vi "LOGIN.vi"() -> ()   [LabVIEW 2020]
uses:
  <vilib>/Utility/file.llb/Read Delimited Spreadsheet (string).vi
  <vilib>/Utility/file.llb/Write Delimited Spreadsheet (string).vi
panel:
  in  "Tab control 2":T1(tab)
  in  "Avanzar 2":bool
  in  "LOGIN 2":bool
  in  "CONTRASEÑA 2":string
  in  "USUARIO  2":string
  in  "Usuario a eliminar 2":string
  in  "Usuario nuevo 2":string
  in  "Contraseña nueva 2":string
  in  "Agregar usuario 2":bool
  in  "Terminar sesión admin 2":bool
  in  "Eliminar usuario 2":bool
  out "Base de datos 2":string[][](array[string])=[["Sabastian", "1234"], ["Fabio", "4321"], ["Keimer", "qwer"], ["Jorge", "0987"]]
  in  "Menu2":enum32{"1", "2", "3", "4", "5", "6"}(tab)
  out "Led8 2":bool
  out "Led7 2":bool
  out "Led6 2":bool
  out "Led5 2":bool
  out "Led4 2":bool
  out "Led3 2":bool
  out "Led2 2":bool
  out "Led1 2":bool
  out "Gráfica del seno 2":cluster{dbl[], dbl[]}(graph)
  out "Circulo de muerte 2":cluster{dbl[], dbl[]}(graph)
  out "tanque de chamber":dbl(slide) scale=0.0..100.0
  out "Fecha 2":string
  out "Hora 2":string
  out "Mensaje de bienvenida 2":string
  in  "Hora y fecha actual 2":bool
  in  "Llenado de un tanque 2":bool
  in  "Circulo de la muerte 2":bool
  in  "Gráfica del seno 2":bool
  in  "Secuencia de leds 2":bool
  in  "Terminar sesión usuario 2":bool
  in  "Tab control 1":T1(tab)
  in  "Avanzar":bool
  in  "LOGIN":bool
  in  "CONTRASEÑA":string
  in  "USUARIO":string
  in  "Usuario a eliminar":string
  in  "Usuario nuevo":string
  in  "Contraseña nueva":string
  in  "Agregar usuario":bool
  in  "Terminar sesión admin":bool
  in  "Eliminar usuario":bool
  out "Base de datos":string[][](array[string])=[["Sabastian", "1234"], ["Fabio", "4321"], ["Keimer", "qwer"], ["Jorge", "0987"]]
  in  "MenuU":enum32{"1", "2", "3", "4", "5", "6"}(tab)
  out "Led8":bool
  out "Led7":bool
  out "Led6":bool
  out "Led5":bool
  out "Led4":bool
  out "Led3":bool
  out "Led2":bool
  out "Led1":bool
  out "Gráfica del seno":cluster{dbl[], dbl[]}(graph)
  out "Circulo de muerte":cluster{dbl[], dbl[]}(graph)
  out "tanque de chamber":dbl(slide) scale=0.0..100.0
  out "Fecha":string
  out "Hora":string
  out "Mensaje de bienvenida":string
  in  "Hora actual y la fehca":bool
  in  "Llenado de un tanque":bool
  in  "Circulo de la muete":bool
  in  "Gráfica del seno":bool
  in  "Secuencia de leds":bool
  in  "Terminar sesión usuario":bool
  # "Bienvenidos"
  # "Fabio Alberto Figueroa Benitez\n\nNatalia Arenas Londoño\n\nLOGIN"
  # "Página principal"
  # "FYN SERVICES"
  # "LOGIN"
  # "Menú del administrador"
  # "Usuarios"
  # "Contraseñas"
  # "Secuencia de un leds"
  # "Llenado de un tanque chamber"
  # "Hora y fecha actual"
  # "Fecha"
  # "Hora"
  # "Bienvenidos"
  # "Fabio Alberto Figueroa Benitez\n\nNatalia Arenas Londoño\n\nLOGIN"
  # "Página principal"
  # "FYN SERVICES"
  # "LOGIN"
  # "Menú del administrador"
  # "Usuarios"
  # "Contraseñas"
  # "Secuencia de un leds"
  # "Llenado de un tanque chamber"
  # "Hora y fecha actual"
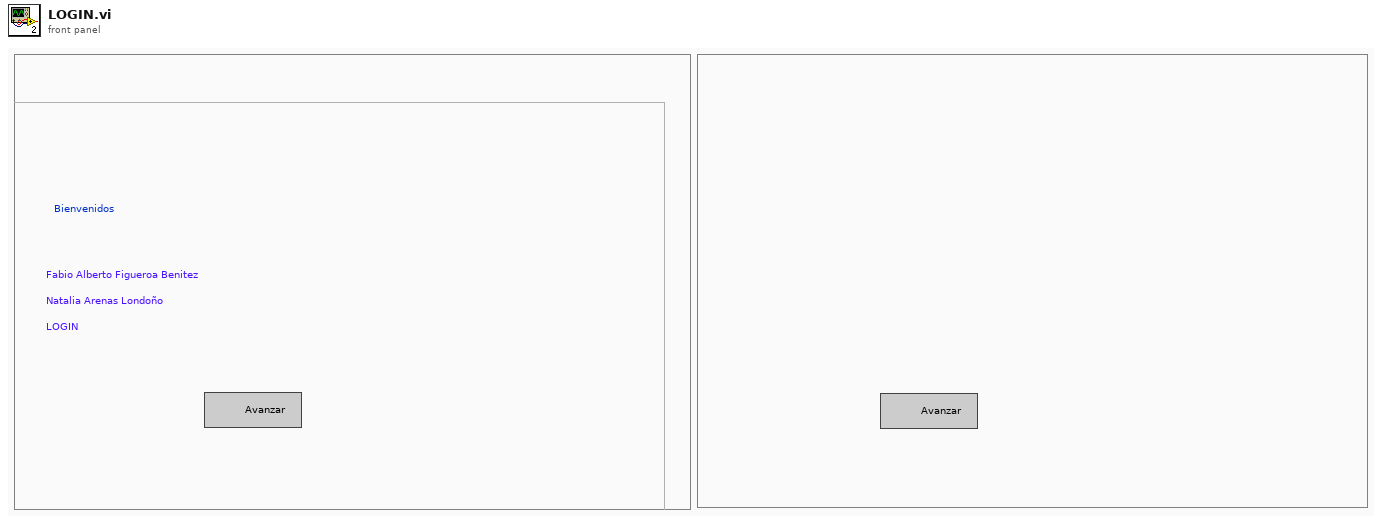
[diagram p1: front panel]
types:
  T1 = enum32{"Bienvenidos", "Principal", "Menú de administrador ", "Menú Usuario"}
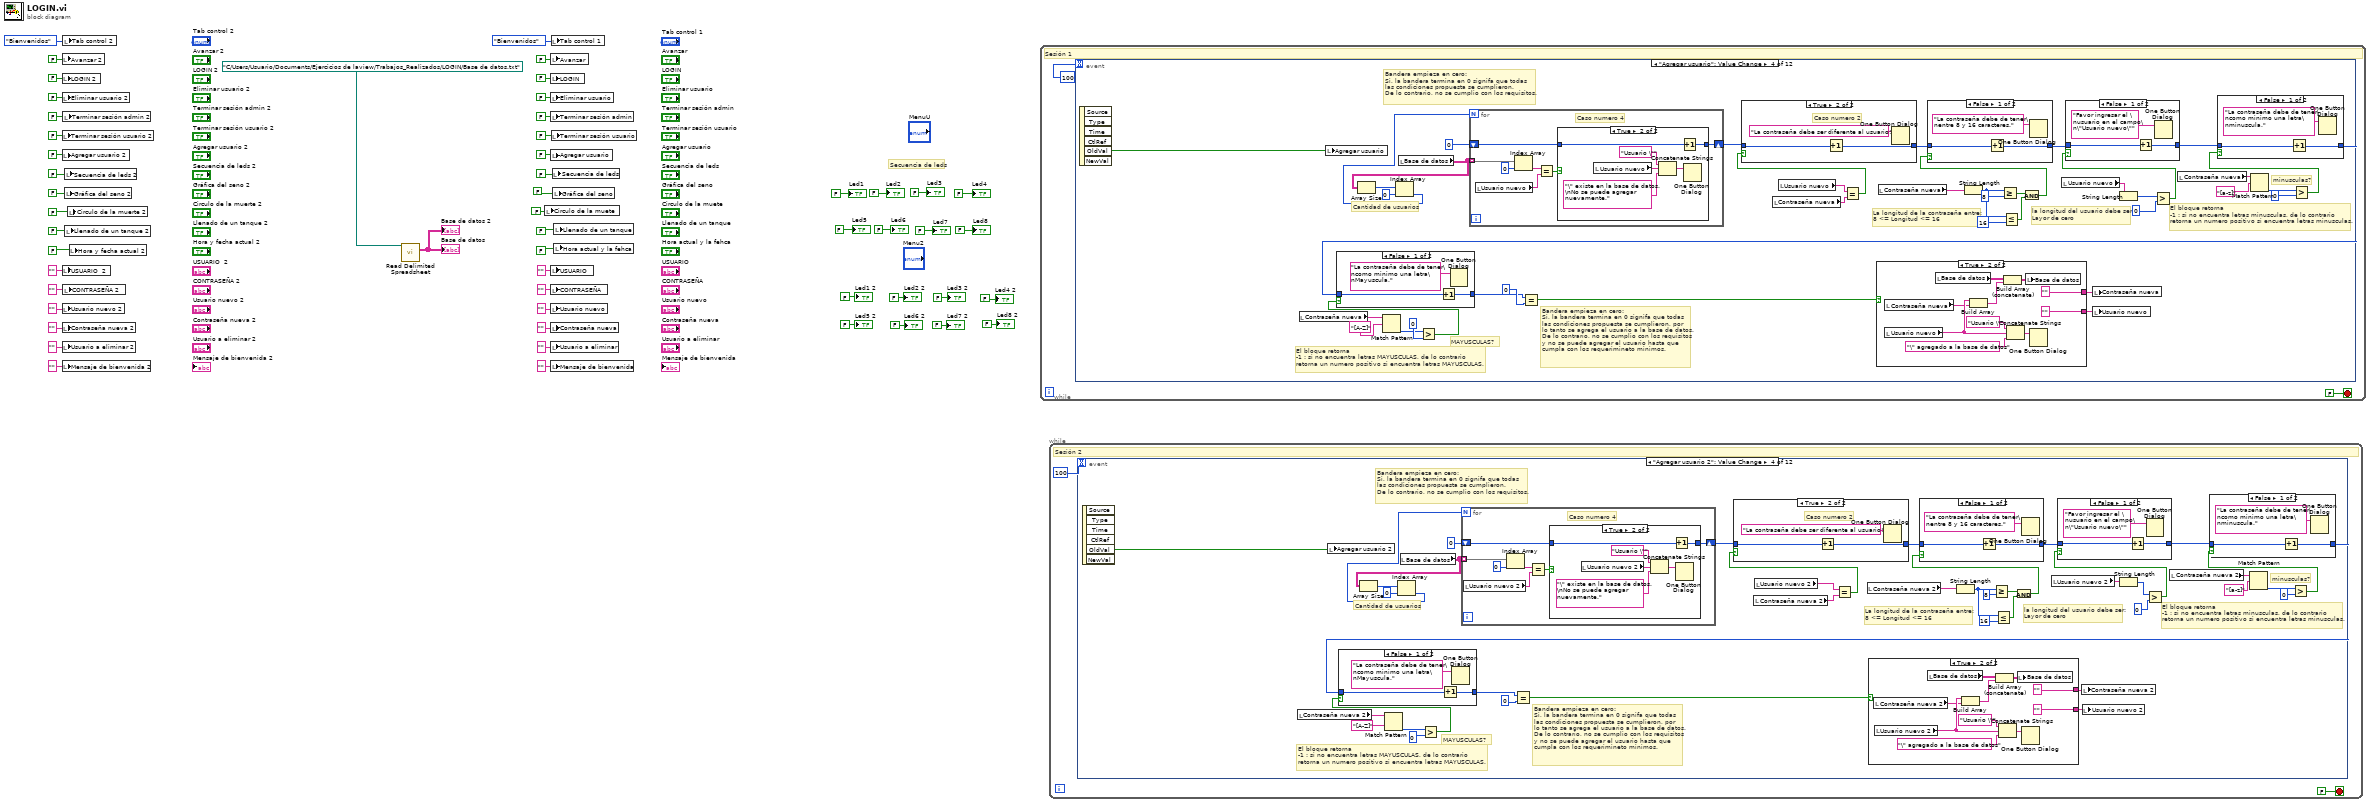
[diagram p0: block diagram]
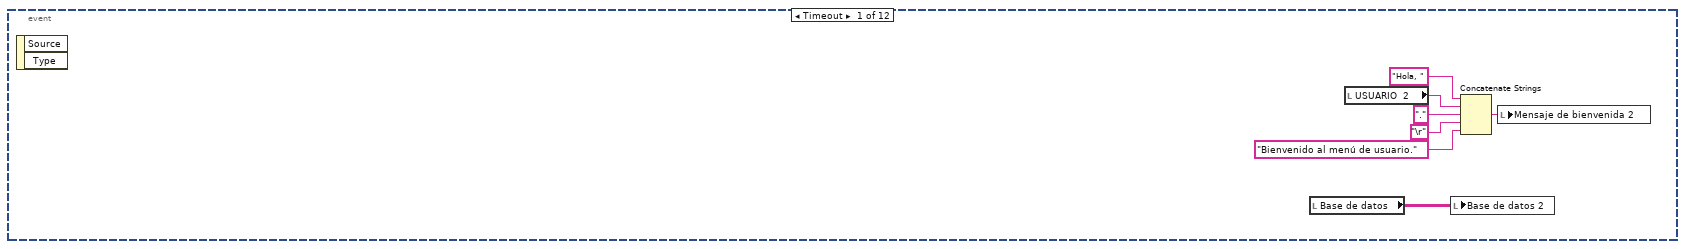
[diagram p2: hidden frame]
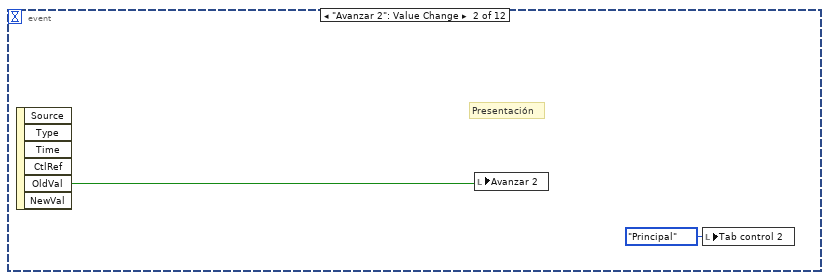
[diagram p3: hidden frame]
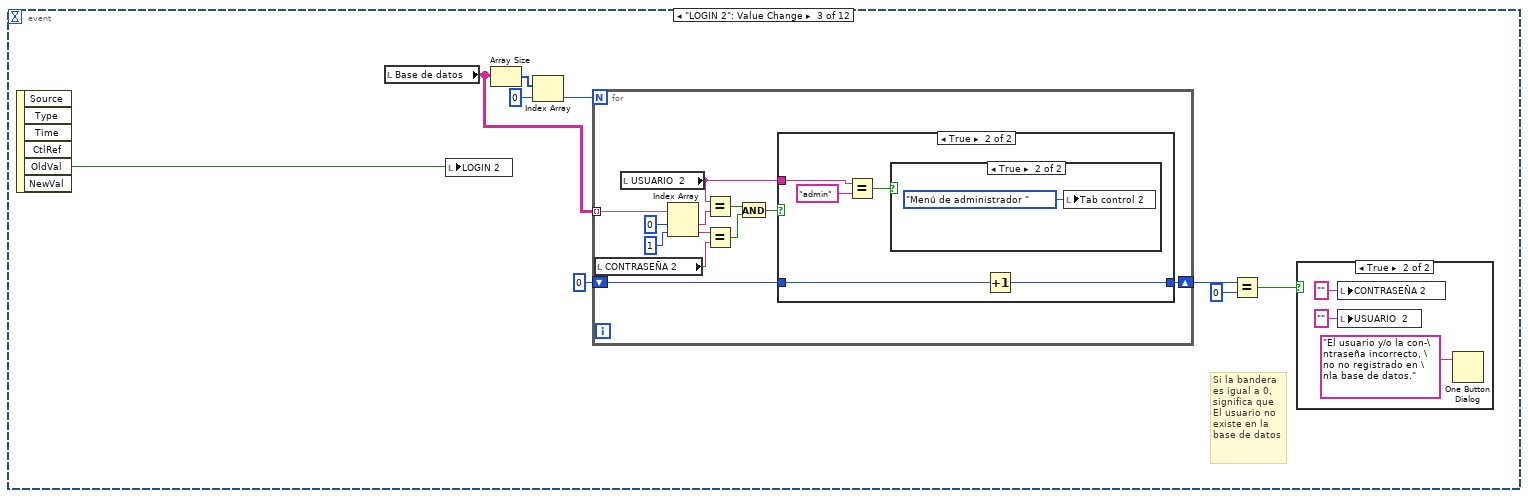
[diagram p4: hidden frame]
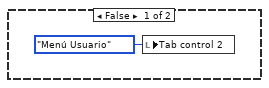
[diagram p7: hidden frame]
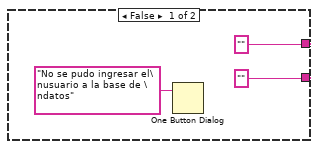
[diagram p8: hidden frame]
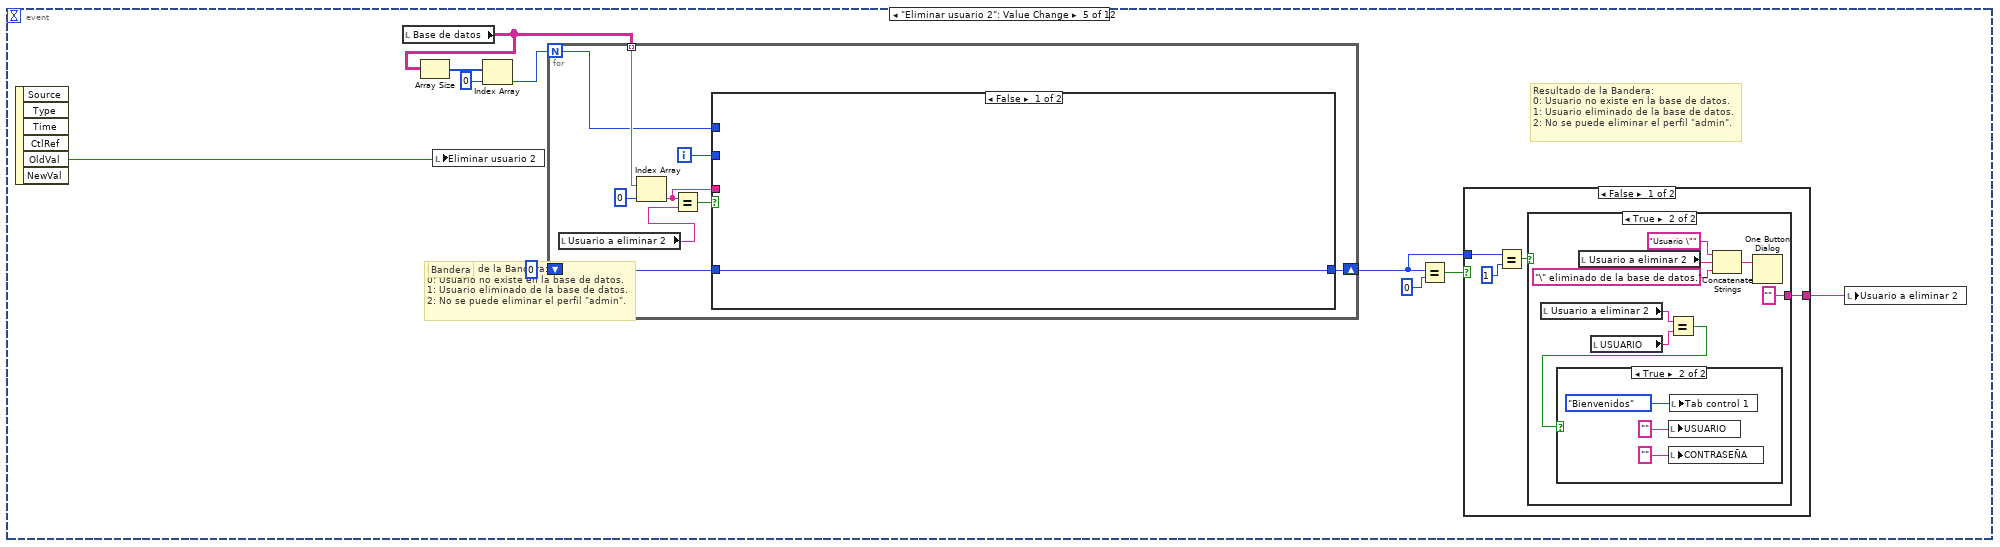
[diagram p15: hidden frame]
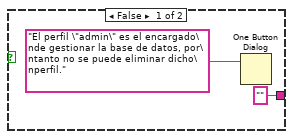
[diagram p16: hidden frame]
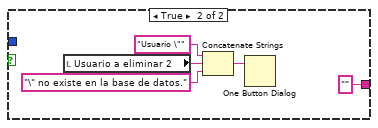
[diagram p18: hidden frame]
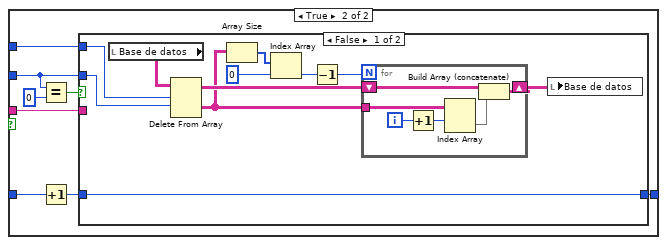
[diagram p19: hidden frame]
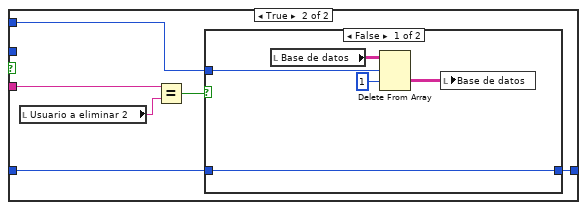
[diagram p20: hidden frame]
diagram:
  # "Secuencia de leds"
  n1 = local write "Avanzar 2"(FALSE ("Avanzar 2")) -> ()
  n2 = local write "LOGIN 2"(FALSE ("LOGIN 2")) -> ()
  n3 = local write "Eliminar usuario 2"(FALSE ("Eliminar usuario 2")) -> ()
  n4 = local write "Terminar sesión usuario 2"(FALSE ("Terminar sesión usuario 2")) -> ()
  n5 = local write "Agregar usuario 2"(FALSE ("Agregar usuario 2")) -> ()
  n6 = local write "USUARIO  2"("" ("USUARIO  2")) -> ()
  n7 = local write "Usuario nuevo 2"("" ("Usuario nuevo 2")) -> ()
  n8 = local write "Contraseña nueva 2"("" ("Contraseña nueva 2")) -> ()
  n9 = local write "Usuario a eliminar 2"("" ("Usuario a eliminar 2")) -> ()
  n10 = local write "Mensaje de bienvenida 2"("" ("Mensaje de bienvenida 2")) -> ()
  n11 = local write "Tab control 2"(T1."Bienvenidos" ("Tab control 2")) -> ()
  n12 = local write "Terminar sesión admin 2"(FALSE ("Terminar sesión admin 2")) -> ()
  n13 = local write "CONTRASEÑA 2"("" ("CONTRASEÑA 2")) -> ()
  n14 = local write "Secuencia de leds 2"(FALSE ("Luces de velocidad variable 2")) -> ()
  n15 = local write "Gráfica del seno 2"(FALSE ("Secuencia de LED 2")) -> ()
  n16 = local write "Llenado de un tanque 2"(FALSE ("Rutina 4 2")) -> ()
  n17 = local write "Circulo de la muerte 2"(FALSE ("Rutina 3 2")) -> ()
  n18 = local write "Hora y fecha actual 2"(FALSE ("Rutina 5 2")) -> ()
  n19 = call-poly <vilib>:"Read Delimited Spreadsheet.vi"("file path (dialog if empty)"=path "C:/Users/Usuario/Documents/Ejercicios de laview/Trabajos_Realizados/LOGIN/Base de datos.txt") -> ("all rows"=→"Base de datos" →"Base de datos 2":string[][])  [unwired: 9 in, 5 out]
  n20 = local write "Circulo de la muete"(FALSE ("Rutina 3")) -> ()
  n21 = local write "Avanzar"(FALSE ("Avanzar")) -> ()
  n22 = local write "LOGIN"(FALSE ("LOGIN")) -> ()
  n23 = local write "Eliminar usuario"(FALSE ("Eliminar usuario")) -> ()
  n24 = local write "Terminar sesión admin"(FALSE ("Terminar sesión admin")) -> ()
  n25 = local write "Agregar usuario"(FALSE ("Agregar usuario")) -> ()
  n26 = local write "USUARIO"("" ("USUARIO")) -> ()
  n27 = local write "CONTRASEÑA"("" ("CONTRASEÑA")) -> ()
  n28 = local write "Usuario nuevo"("" ("Usuario nuevo")) -> ()
  n29 = local write "Contraseña nueva"("" ("Contraseña nueva")) -> ()
  n30 = local write "Usuario a eliminar"("" ("Usuario a eliminar")) -> ()
  n31 = local write "Mensaje de bienvenida"("" ("Mensaje de bienvenida")) -> ()
  n32 = local write "Tab control 1"(T1."Bienvenidos" ("Tab control 1")) -> ()
  n33 = local write "Terminar sesión usuario"(FALSE ("Terminar sesión usuario")) -> ()
  n34 = local write "Secuencia de leds"(FALSE ("Luces de velocidad variable")) -> ()
  n35 = local write "Gráfica del seno"(FALSE ("Secuencia de LED")) -> ()
  n36 = local write "Llenado de un tanque"(FALSE ("Rutina 4")) -> ()
  n37 = local write "Hora actual y la fehca"(FALSE ("Rutina 5")) -> ()
  n38 = while {
    stop <- FALSE stop-if-true
    # "Sesión 1"
    n39 = event shown="[3] \"Agregar usuario\": Value Change" {
      selector: _ -> [_ _ _ _ _ _ _ _ _ _ _ _]
      dyn-events: _ -> [_ _ _ _ _ _ _ _ _ _ _ _]
      timeout: 100 -> [_ _ _ _ _ _ _ _ _ _ _ _]
      event Timeout {
        n40 = event-data() -> ()  [unwired: 1 in, 2 out]
        n41 = local read "Base de datos"() -> (w58:string[][])
        n42 = call-poly <vilib>:"Write Delimited Spreadsheet.vi"("file path (dialog if empty)"=path "C:/Users/Usuario/Documents/Ejercicios de laview/Trabajos_Realizados/LOGIN/Base de datos.txt", "2D data"=w58, "append to file? (new file:F)"=FALSE) -> ()  [unwired: 11 in, 2 out]
        n43 = local read "USUARIO"() -> (w64:string)
        n44 = Concatenate Strings("Hola, ", w64, ".", "\r", "Bienvenido al menú de usuario.") -> (w62:string)
        n45 = local write "Mensaje de bienvenida"(w62) -> ()
      }
      event "Avanzar": Value Change {
        # "Presentación"
        n46 = event-data() -> ("OldVal"=w66:bool)  [unwired: 1 in, 5 out]
        n47 = local write "Avanzar"(w66) -> ()
        n48 = local write "Tab control 1"(T1."Principal" ("Tab control")) -> ()
      }
      event "LOGIN": Value Change {
        # "Si la bandera \nes igual a 0,\nsignifica que\nEl usuario no \nexiste en la \nbase de datos"
        n49 = event-data() -> ("OldVal"=w76:bool)  [unwired: 1 in, 5 out]
        n50 = local write "LOGIN"(w76) -> ()
        n51 = local read "Base de datos"() -> (w72:string[][])
        n52 = Array Size(array=w72) -> (size(s)=w74:i32[])
        n53 = Index Array(array=w74, index=0) -> (element=w73:i32)
        n54 = for {
          N: w73 -> [_]
          tunnel: w72 -> [w91] mode=indexing
          shift-right: [w80] -> w70
          shift-left: 0 -> [w81]
          n55 = local read "CONTRASEÑA"() -> (w86:string)
          n56 = local read "USUARIO"() -> (w82:string)
          n57 = Index Array(array=w91, index #1=0 ("index"), index #2=1 ("index")) -> (element #1=w88:string, element #2=w87:string)
          n58 = Equal?(x=w82, y=w88) -> (x = y?=w85:bool)
          n59 = Equal?(x=w87, y=w86) -> (x = y?=w84:bool)
          n60 = And(x=w85, y=w84) -> (x .and. y?=w83:bool)
          n61 = case shown="True" w83 {
            tunnel: w82 -> [_ w97]
            tunnel: w81 -> [w92 w94]
            tunnel: [w92 w93] -> w80
            frame False {
            }
            frame True {
              n62 = Equal?(x=w97, y="admin") -> (x = y?=w95:bool)
              n63 = case shown="False" w95 {
                frame False {
                  n64 = local write "Tab control 1"(T1."Menú Usuario" ("Tab control")) -> ()
                }
                frame True {
                  n65 = local write "Tab control 1"(T1."Menú de administrador " ("Tab control")) -> ()
                }
              }
              n66 = Increment(x=w94) -> (x+1=w93:i32)
            }
          }
        }
        n67 = Equal?(x=w70, y=0) -> (x = y?=w68:bool)
        n68 = case shown="True" w68 {
          frame False {
          }
          frame True {
            n69 = local write "CONTRASEÑA"("") -> ()
            n70 = local write "USUARIO"("") -> ()
            n71 = One Button Dialog(message="El usuario y/o la con-\ntraseña incorrecto, \no no registrado en \nla base de datos.") -> ()  [unwired: 1 in, 1 out]
          }
        }
      }
      event "Agregar usuario": Value Change {
        # "Bandera empieza en cero:\nSi, la bandera termina en 0 signifa que todas \nlas condiciones propuesta se cumplieron, por \nlo tanto se agrega el usuario a la base de datos.\nDe lo contrario, no se cumplio con los requisitos\ny no se puede agregar el usuario hasta que \ncumpla con los requerimineto minimos."
        # "MAYUSCULAS?"
        # "El bloque retorna \n-1 : si no encuentra letras MAYUSCULAS, de lo contrario\nretorna un numero positivo si encuentra letras MAYUSCULAS."
        # "minusculas?"
        # "El bloque retorna \n-1 : si no encuentra letras minusculas, de lo contrario\nretorna un numero positivo si encuentra letras minusculas."
        # "la longitud del usuario debe ser:\nLayor de cero"
        # "La longitud de la contraseña entre:\n8 <= Longitud <= 16"
        # "Cantidad de usuarios"
        # "Bandera empieza en cero:\nSi, la bandera termina en 0 signifa que todas \nlas condiciones propuesta se cumplieron.\nDe lo contrario, no se cumplio con los requisitos."
        n72 = event-data() -> ("OldVal"=w139:bool)  [unwired: 1 in, 5 out]
        n73 = local read "Contraseña nueva"() -> (w107:string)
        n74 = local write "Agregar usuario"(w139) -> ()
        n75 = Match Pattern(string=w107, regular expression="[A-Z]") -> (offset past match=w110:i32)  [unwired: 1 in, 3 out]
        n76 = local read "Base de datos"() -> (w135:string[][])
        n77 = Array Size(array=w135) -> (size(s)=w137:i32[])
        n78 = Index Array(array=w137, index=0) -> (element=w134:i32)
        n79 = Greater?(x=w110, y=0) -> (0:w106:bool)
        n80 = for {
          N: w134 -> [_]
          tunnel: w135 -> [w178] mode=indexing
          shift-right: [w173] -> w131
          shift-left: 0 -> [w174]
          # "Caso numero 4"
          n81 = local read "Usuario nuevo"() -> (w176:string)
          n82 = Index Array(array=w178, index=0) -> (element=w177:string)
          n83 = Equal?(x=w177, y=w176) -> (x = y?=w175:bool)
          n84 = case shown="True" w175 {
            tunnel: w174 -> [w180 w182]
            tunnel: [w180 w181] -> w173
            frame False {
            }
            frame True {
              n85 = local read "Usuario nuevo"() -> (w183:string)
              n86 = Concatenate Strings("Usuario \"", w183, "\" existe en la base de datos.\nNo se puede agregar nuevamente." ("message")) -> (w185:string)
              n87 = Increment(x=w182) -> (x+1=w181:i32)
              n88 = One Button Dialog(message=w185) -> ()  [unwired: 1 in, 1 out]
            }
          }
        }
        n89 = local read "Contraseña nueva"() -> (w133:string)
        n90 = local read "Usuario nuevo"() -> (w132:string)
        n91 = Equal?(x=w132, y=w133) -> (x = y?=w100:bool)
        n92 = case shown="True" w100 {
          tunnel: w131 -> [w169 w170]
          tunnel: [w169 w171] -> w126
          frame False {
          }
          frame True {
            # "Caso numero 2"
            n93 = Increment(x=w170) -> (x+1=w171:i32)
            n94 = One Button Dialog(message="La contraseña debe ser diferente al usuario!") -> ()  [unwired: 1 in, 1 out]
          }
        }
        n95 = local read "Contraseña nueva"() -> (w124:string)
        n96 = String Length(string=w124) -> (length=w125:i32)
        n97 = Greater Or Equal?(x=w125, y=8) -> (x >= y?=w128:bool)
        n98 = Less Or Equal?(x=w125, y=16) -> (x <= y?=w127:bool)
        n99 = And(x=w128, y=w127) -> (x .and. y?=w123:bool)
        n100 = case shown="False" w123 {
          tunnel: w126 -> [w165 w168]
          tunnel: [w167 w168] -> w120
          frame False {
            n101 = Increment(x=w165) -> (x+1=w167:i32)
            n102 = One Button Dialog(message="La contraseña debe de tener\nentre 8 y 16 caracteres.") -> ()  [unwired: 1 in, 1 out]
          }
          frame True {
          }
        }
        n103 = local read "Usuario nuevo"() -> (w119:string)
        n104 = String Length(string=w119) -> (length=w122:i32)
        n105 = Greater?(x=w122, y=0) -> (0:w118:bool)
        n106 = case shown="False" w118 {
          tunnel: w120 -> [w163 w164]
          tunnel: [w162 w164] -> w114
          frame False {
            n107 = Increment(x=w163) -> (x+1=w162:i32)
            n108 = One Button Dialog(message="Favor ingresar el \nusuario en el campo\n\"Usuario nuevo\"") -> ()  [unwired: 1 in, 1 out]
          }
          frame True {
          }
        }
        n109 = local read "Contraseña nueva"() -> (w112:string)
        n110 = Match Pattern(string=w112, regular expression="[a-z]") -> (offset past match=w116:i32)  [unwired: 1 in, 3 out]
        n111 = Greater?(x=w116, y=0) -> (0:w113:bool)
        n112 = case shown="False" w113 {
          tunnel: w114 -> [w157 w160]
          tunnel: [w159 w160] -> w108
          frame False {
            n113 = Increment(x=w157) -> (x+1=w159:i32)
            n114 = One Button Dialog(message="La contraseña debe de tener\ncomo minimo una letra\nminuscula.") -> ()  [unwired: 1 in, 1 out]
          }
          frame True {
          }
        }
        n115 = case shown="False" w106 {
          tunnel: w108 -> [w153 w156]
          tunnel: [w155 w156] -> w104
          frame False {
            n116 = Increment(x=w153) -> (x+1=w155:i32)
            n117 = One Button Dialog(message="La contraseña debe de tener\ncomo minimo una letra\nMayuscula.") -> ()  [unwired: 1 in, 1 out]
          }
          frame True {
          }
        }
        n118 = Equal?(x=w104, y=0) -> (x = y?=w103:bool)
        n119 = case shown="True" w103 {
          tunnel: ["" ""] -> w102
          tunnel: ["" ""] -> w101
          frame False {
            n120 = One Button Dialog(message="No se pudo ingresar el\nusuario a la base de \ndatos") -> ()  [unwired: 1 in, 1 out]
          }
          frame True {
            n121 = local read "Contraseña nueva"() -> (w145:string)
            n122 = local read "Usuario nuevo"() -> (w146:string)
            n123 = local read "Base de datos"() -> (w147:string[][])
            n124 = Build Array(w146, w145) -> (w150:string[])
            n125 = Build Array (concatenate)(w147, w150) -> (w151:string[][])
            n126 = Concatenate Strings("Usuario \"", w146, "\" agregado a la base de datos" ("message")) -> (w152:string)
            n127 = local write "Base de datos"(w151) -> ()
            n128 = One Button Dialog(message=w152) -> ()  [unwired: 1 in, 1 out]
          }
        }
        n129 = local write "Contraseña nueva"(w102) -> ()
        n130 = local write "Usuario nuevo"(w101) -> ()
      }
      event "Eliminar usuario": Value Change {
        # "Resultado de la Bandera:\n0: Usuario no existe en la base de datos.\n1: Usuario eliminado de la base de datos.\n2: No se puede eliminar el perfil \"admin\"."
        # "Bandera"
        # "Resultado de la Bandera:\n0: Usuario no existe en la base de datos.\n1: Usuario eliminado de la base de datos.\n2: No se puede eliminar el perfil \"admin\"."
        n131 = event-data() -> ("OldVal"=w196:bool)  [unwired: 1 in, 5 out]
        n132 = local write "Eliminar usuario"(w196) -> ()
        n133 = local read "Base de datos"() -> (w192:string[][])
        n134 = Array Size(array=w192) -> (size(s)=w195:i32[])
        n135 = Index Array(array=w195, index=0) -> (element=w193:i32)
        n136 = for {
          N: w193 -> [w222]
          tunnel: w192 -> [w226] mode=indexing
          shift-right: [w220] -> w188
          shift-left: 0 -> [w221]
          i -> [w223]
          n137 = local read "Usuario a eliminar"() -> (w225:string)
          n138 = Index Array(array=w226, index=0) -> (element=w219:string)
          n139 = Equal?(x=w219, y=w225) -> (x = y?=w224:bool)
          n140 = case shown="True" w224 {
            tunnel: w223 -> [_ w233]
            tunnel: w222 -> [_ w234]
            tunnel: w221 -> [w228 w231]
            tunnel: [w228 w229] -> w220
            tunnel: w219 -> [_ w232]
            frame False {
            }
            frame True {
              n141 = Equal?(x=w233, y=0) -> (x = y?=w235:bool)
              n142 = Increment(x=w231) -> (x+1=w230:i32)
              n143 = case shown="False" w235 {
                tunnel: w234 -> [w243 w256]
                tunnel: w233 -> [w242 _]
                tunnel: w232 -> [_ w258]
                tunnel: w230 -> [w237 w255]
                tunnel: [w237 w254] -> w229
                frame False {
                  n144 = local read "Base de datos"() -> (w244:string[][])
                  n145 = Delete From Array(array=w244, length=w243, index (row)=w242) -> (deleted portion=w239:string[][], array with subset deleted=w240:string[][])  [unwired: 1 in]
                  n146 = Array Size(array=w239) -> (size(s)=w246:i32[])
                  n147 = Index Array(array=w246, index=0) -> (element=w245:i32)
                  n148 = Decrement(x=w245) -> (x-1=w241:i32)
                  n149 = for {
                    N: w241 -> [_]
                    shift-right: [w248] -> w238
                    shift-left: w240 -> [w252]
                    tunnel: w239 -> [w251]
                    i -> [w253]
                    n150 = Increment(x=w253) -> (x+1=w250:i32)
                    n151 = Index Array(array=w251, index (row)=w250) -> (element=w249:string[])  [unwired: 1 in]
                    n152 = Build Array (concatenate)(w252, w249) -> (w248:string[][])
                  }
                  n153 = local write "Base de datos"(w238) -> ()
                }
                frame True {
                  n154 = local read "Usuario a eliminar"() -> (w259:string)
                  n155 = Equal?(x=w258, y=w259) -> (x = y?=w257:bool)
                  n156 = case shown="True" w257 {
                    tunnel: w256 -> [w261 _]
                    tunnel: w255 -> [w260 w266]
                    tunnel: [w260 w265] -> w254
                    frame False {
                      n157 = local read "Base de datos"() -> (w264:string[][])
                      n158 = Delete From Array(array=w264, length=w261, index (row)=1) -> (deleted portion=w263:string[][])  [unwired: 1 in, 1 out]
                      n159 = local write "Base de datos"(w263) -> ()
                    }
                    frame True {
                      n160 = Increment(x=w266) -> (x+1=w265:i32)
                      n161 = One Button Dialog(message="No se puede eliminar el perfir de \"admin\".") -> ()  [unwired: 1 in, 1 out]
                    }
                  }
                }
              }
            }
          }
        }
        n162 = Equal?(x=w188, y=0) -> (x = y?=w189:bool)
        n163 = case shown="False" w189 {
          tunnel: w188 -> [w199 _]
          tunnel: [w197 ""] -> w187
          frame False {
            n164 = Equal?(x=w199, y=1) -> (x = y?=w200:bool)
            n165 = case shown="True" w200 {
              tunnel: ["" ""] -> w197
              frame False {
                n166 = One Button Dialog(message="El perfil \"admin\" es el encargado\nde gestionar la base de datos, por\ntanto no se puede eliminar dicho\nperfil.") -> ()  [unwired: 1 in, 1 out]
              }
              frame True {
                n167 = local read "Usuario a eliminar"() -> (w204:string)
                n168 = local read "USUARIO  2"() -> (w205:string)
                n169 = local read "Usuario a eliminar"() -> (w209:string)
                n170 = Equal?(x=w204, y=w205) -> (x = y?=w203:bool)
                n171 = case shown="True" w203 {
                  frame False {
                  }
                  frame True {
                    n172 = local write "USUARIO  2"("") -> ()
                    n173 = local write "Tab control 2"(T1."Bienvenidos" ("Tab control")) -> ()
                    n174 = local write "CONTRASEÑA 2"("") -> ()
                  }
                }
                n175 = Concatenate Strings("Usuario \"", w209, "\" eliminado de la base de datos." ("message")) -> (w210:string)
                n176 = One Button Dialog(message=w210) -> ()  [unwired: 1 in, 1 out]
              }
            }
          }
          frame True {
            n177 = local read "Usuario a eliminar"() -> (w215:string)
            n178 = Concatenate Strings("Usuario \"", w215, "\" no existe en la base de datos." ("message")) -> (w218:string)
            n179 = One Button Dialog(message=w218) -> ()  [unwired: 1 in, 1 out]
          }
        }
        n180 = local write "Usuario a eliminar"(w187) -> ()
      }
      event "Terminar sesión admin": Value Change {
        n181 = event-data() -> ("OldVal"=w271:bool)  [unwired: 1 in, 5 out]
        n182 = local write "Terminar sesión admin"(w271) -> ()
        n183 = local write "Tab control 1"(T1."Bienvenidos" ("Tab control")) -> ()
        n184 = local write "USUARIO"("") -> ()
        n185 = local write "CONTRASEÑA"("") -> ()
      }
      event "Terminar sesión usuario": Value Change {
        n186 = event-data() -> ("OldVal"=w272:bool)  [unwired: 1 in, 5 out]
        n187 = local write "Terminar sesión usuario"(w272) -> ()
        n188 = local write "Tab control 1"(T1."Bienvenidos" ("Tab control")) -> ()
        n189 = local write "USUARIO"("") -> ()
        n190 = local write "CONTRASEÑA"("") -> ()
      }
      event "Secuencia de leds": Value Change {
        # "Secuencia de leds"
        n191 = event-data() -> ("OldVal"=w277:bool)  [unwired: 1 in, 5 out]
        n192 = local write "Secuencia de leds"(w277) -> ()
        n193 = flat-sequence {
          frame #0 {
            n194 = local read "Led1"() -> (w280:bool)
            n195 = Not(x=w280) -> (.not. x?=w279:bool)
            n196 = Wait (ms)(milliseconds to wait=u32 1000) -> ()  [unwired: 1 out]
            n197 = local write "Led1"(w279) -> ()
          }
          frame #1 {
            n198 = local read "Led2"() -> (w282:bool)
            n199 = Wait (ms)(milliseconds to wait=u32 1000) -> ()  [unwired: 1 out]
            n200 = Not(x=w282) -> (.not. x?=w283:bool)
            n201 = local write "Led2"(w283) -> ()
            n202 = local write "Led1"(FALSE ("Led1")) -> ()
          }
          frame #2 {
            n203 = local read "Led3"() -> (w287:bool)
            n204 = Wait (ms)(milliseconds to wait=u32 1000) -> ()  [unwired: 1 out]
            n205 = Not(x=w287) -> (.not. x?=w286:bool)
            n206 = local write "Led3"(w286) -> ()
            n207 = local write "Led2"(FALSE ("Led1")) -> ()
          }
          frame #3 {
            n208 = local read "Led4"() -> (w291:bool)
            n209 = Wait (ms)(milliseconds to wait=u32 1000) -> ()  [unwired: 1 out]
            n210 = Not(x=w291) -> (.not. x?=w292:bool)
            n211 = local write "Led4"(w292) -> ()
            n212 = local write "Led3"(FALSE ("Led1")) -> ()
          }
          frame #4 {
            n213 = local read "Led5"() -> (w294:bool)
            n214 = Wait (ms)(milliseconds to wait=u32 1000) -> ()  [unwired: 1 out]
            n215 = Not(x=w294) -> (.not. x?=w293:bool)
            n216 = local write "Led5"(w293) -> ()
            n217 = local write "Led4"(FALSE ("Led1")) -> ()
          }
          frame #5 {
            n218 = local read "Led6"() -> (w299:bool)
            n219 = Wait (ms)(milliseconds to wait=u32 1000) -> ()  [unwired: 1 out]
            n220 = Not(x=w299) -> (.not. x?=w300:bool)
            n221 = local write "Led6"(w300) -> ()
            n222 = local write "Led5"(FALSE ("Led1")) -> ()
          }
          frame #6 {
            n223 = local read "Led7"() -> (w303:bool)
            n224 = Wait (ms)(milliseconds to wait=u32 1000) -> ()  [unwired: 1 out]
            n225 = Not(x=w303) -> (.not. x?=w302:bool)
            n226 = local write "Led7"(w302) -> ()
            n227 = local write "Led6"(FALSE ("Led1")) -> ()
          }
          frame #7 {
            n228 = local read "Led8"() -> (w306:bool)
            n229 = Wait (ms)(milliseconds to wait=u32 1000) -> ()  [unwired: 1 out]
            n230 = Not(x=w306) -> (.not. x?=w307:bool)
            n231 = local write "Led8"(w307) -> ()
            n232 = local write "Led7"(FALSE ("Led1")) -> ()
          }
          frame #8 {
            n233 = Wait (ms)(milliseconds to wait=u32 1000) -> ()  [unwired: 1 out]
            n234 = local write "Led8"(FALSE ("Led1")) -> ()
          }
        }
        n235 = local write "MenuU"(enum32{"1", "2", "3", "4", "5", "6"}."2" ("MenuU")) -> ()
      }
      event "Gráfica del seno": Value Change {
        # "Gráfica del seno"
        # "Este bloque\nrecibe un cluster"
        # "Para mostrar la gráfoca en x,  y"
        n236 = event-data() -> ("OldVal"=w311:bool)  [unwired: 1 in, 5 out]
        n237 = local write "MenuU"(enum32{"1", "2", "3", "4", "5", "6"}."3" ("MenuU")) -> ()
        n238 = local write "Gráfica del seno"(w311) -> ()
        n239 = Multiply(x=200.0, y=3.141592653589793) -> (x*y=w317:dbl)
        n240 = for {
          N: w317 -> [_]
          tunnel: [w320] -> w312 mode=indexing
          tunnel: [w319] -> w313 mode=indexing
          i -> [w323]
          # "x"
          # "y"
          n241 = Wait (ms)(milliseconds to wait=u32 1) -> ()  [unwired: 1 out]
          n242 = Divide(x=w323, y=100) -> (x/y=w319:dbl)
          n243 = Sine(x=w319) -> (sin(x)=w320:dbl)
        }
        n244 = Bundle(w313, w312) -> (→"Gráfica del seno":cluster{dbl[], dbl[]})  [unwired: 1 in]
      }
      event "Circulo de la muete": Value Change {
        n245 = event-data() -> ("OldVal"=w329:bool)  [unwired: 1 in, 5 out]
        n246 = local write "Circulo de la muete"(w329) -> ()
        n247 = for {
          N: 100 -> [_]
          tunnel: [w332] -> w327 mode=indexing
          tunnel: [w330] -> w326 mode=indexing
          i -> [w331]
          n248 = Multiply(x=0.3183098861837907, y=w331) -> (x*y=w334:dbl)
          n249 = Sine & Cosine(0:w334) -> (1:w333:dbl, 2:w330:dbl)
          n250 = Multiply(x=w333, y=w331) -> (x*y=w332:dbl)
        }
        n251 = local write "MenuU"(enum32{"1", "2", "3", "4", "5", "6"}."4" ("MenuU")) -> ()
        n252 = Bundle(w327, w326) -> (→"Circulo de muerte":cluster{dbl[], dbl[]})  [unwired: 1 in]
      }
      event "Llenado de un tanque": Value Change {
        n253 = event-data() -> ("OldVal"=w338:bool)  [unwired: 1 in, 5 out]
        n254 = local write "Llenado de un tanque"(w338) -> ()
        n255 = for {
          N: 100 -> [_]
          i -> [w340]
          n256 = Wait (ms)(milliseconds to wait=u32 100) -> ()  [unwired: 1 out]
          "tanque de chamber" <- w340
        }
        n257 = local write "MenuU"(enum32{"1", "2", "3", "4", "5", "6"}."5" ("MenuU")) -> ()
      }
      event "Hora actual y la fehca": Value Change {
        # "Hora"
        # "Fecha"
        n258 = event-data() -> ("OldVal"=w353:bool)  [unwired: 1 in, 5 out]
        n259 = local write "Hora actual y la fehca"(w353) -> ()
        n260 = Get Date/Time In Seconds() -> (seconds since 1Jan1904=w352:timestamp)
        n261 = Get Date/Time In Seconds() -> (seconds since 1Jan1904=w342:timestamp)
        n262 = local write "MenuU"(enum32{"1", "2", "3", "4", "5", "6"}."6" ("MenuU")) -> ()
        n263 = Get Date/Time String(seconds (now)=w352) -> (date string=w351:string)  [unwired: 2 in, 1 out]
        n264 = Get Date/Time String(seconds (now)=w342) -> (time string=w341:string)  [unwired: 2 in, 1 out]
        n265 = Concatenate Strings("Fecha:" ("date string"), "\n", "\n", w351) -> (→"Fecha":string)
        n266 = Concatenate Strings("Hora:" ("date string"), "\n", "\n", w341) -> (→"Hora":string)
      }
    }
  }
  n267 = while {
    stop <- FALSE stop-if-true
    # "Sesión 2"
    n268 = event shown="[3] \"Agregar usuario 2\": Value Change" {
      selector: _ -> [_ _ _ _ _ _ _ _ _ _ _ _]
      dyn-events: _ -> [_ _ _ _ _ _ _ _ _ _ _ _]
      timeout: 100 -> [_ _ _ _ _ _ _ _ _ _ _ _]
      event Timeout {
        n269 = event-data() -> ()  [unwired: 1 in, 2 out]
        n270 = local read "Base de datos"() -> (w357:string[][])
        n271 = local read "USUARIO  2"() -> (w362:string)
        n272 = local write "Base de datos 2"(w357) -> ()
        n273 = Concatenate Strings("Hola, ", w362, ".", "\r", "Bienvenido al menú de usuario.") -> (w360:string)
        n274 = local write "Mensaje de bienvenida 2"(w360) -> ()
      }
      event "Avanzar 2": Value Change {
        # "Presentación"
        n275 = event-data() -> ("OldVal"=w364:bool)  [unwired: 1 in, 5 out]
        n276 = local write "Avanzar 2"(w364) -> ()
        n277 = local write "Tab control 2"(T1."Principal" ("Tab control")) -> ()
      }
      event "LOGIN 2": Value Change {
        # "Si la bandera \nes igual a 0,\nsignifica que\nEl usuario no \nexiste en la \nbase de datos"
        n278 = event-data() -> ("OldVal"=w374:bool)  [unwired: 1 in, 5 out]
        n279 = local read "Base de datos"() -> (w370:string[][])
        n280 = local write "LOGIN 2"(w374) -> ()
        n281 = Array Size(array=w370) -> (size(s)=w372:i32[])
        n282 = Index Array(array=w372, index=0) -> (element=w371:i32)
        n283 = for {
          N: w371 -> [_]
          tunnel: w370 -> [w389] mode=indexing
          shift-right: [w378] -> w368
          shift-left: 0 -> [w379]
          n284 = local read "CONTRASEÑA 2"() -> (w384:string)
          n285 = local read "USUARIO  2"() -> (w380:string)
          n286 = Index Array(array=w389, index #1=0 ("index"), index #2=1 ("index")) -> (element #1=w386:string, element #2=w385:string)
          n287 = Equal?(x=w380, y=w386) -> (x = y?=w383:bool)
          n288 = Equal?(x=w385, y=w384) -> (x = y?=w382:bool)
          n289 = And(x=w383, y=w382) -> (x .and. y?=w381:bool)
          n290 = case shown="True" w381 {
            tunnel: w380 -> [_ w395]
            tunnel: w379 -> [w390 w392]
            tunnel: [w390 w391] -> w378
            frame False {
            }
            frame True {
              n291 = Equal?(x=w395, y="admin") -> (x = y?=w393:bool)
              n292 = case shown="True" w393 {
                frame False {
                  n293 = local write "Tab control 2"(T1."Menú Usuario" ("Tab control")) -> ()
                }
                frame True {
                  n294 = local write "Tab control 2"(T1."Menú de administrador " ("Tab control")) -> ()
                }
              }
              n295 = Increment(x=w392) -> (x+1=w391:i32)
            }
          }
        }
        n296 = Equal?(x=w368, y=0) -> (x = y?=w366:bool)
        n297 = case shown="True" w366 {
          frame False {
          }
          frame True {
            n298 = local write "CONTRASEÑA 2"("") -> ()
            n299 = local write "USUARIO  2"("") -> ()
            n300 = One Button Dialog(message="El usuario y/o la con-\ntraseña incorrecto, \no no registrado en \nla base de datos.") -> ()  [unwired: 1 in, 1 out]
          }
        }
      }
      event "Agregar usuario 2": Value Change {
        # "Bandera empieza en cero:\nSi, la bandera termina en 0 signifa que todas \nlas condiciones propuesta se cumplieron, por \nlo tanto se agrega el usuario a la base de datos.\nDe lo contrario, no se cumplio con los requisitos\ny no se puede agregar el usuario hasta que \ncumpla con los requerimineto minimos."
        # "MAYUSCULAS?"
        # "El bloque retorna \n-1 : si no encuentra letras MAYUSCULAS, de lo contrario\nretorna un numero positivo si encuentra letras MAYUSCULAS."
        # "minusculas?"
        # "El bloque retorna \n-1 : si no encuentra letras minusculas, de lo contrario\nretorna un numero positivo si encuentra letras minusculas."
        # "la longitud del usuario debe ser:\nLayor de cero"
        # "La longitud de la contraseña entre:\n8 <= Longitud <= 16"
        # "Cantidad de usuarios"
        # "Bandera empieza en cero:\nSi, la bandera termina en 0 signifa que todas \nlas condiciones propuesta se cumplieron.\nDe lo contrario, no se cumplio con los requisitos."
        n301 = event-data() -> ("OldVal"=w437:bool)  [unwired: 1 in, 5 out]
        n302 = local read "Contraseña nueva 2"() -> (w405:string)
        n303 = local write "Agregar usuario 2"(w437) -> ()
        n304 = Match Pattern(string=w405, regular expression="[A-Z]") -> (offset past match=w408:i32)  [unwired: 1 in, 3 out]
        n305 = local read "Base de datos"() -> (w433:string[][])
        n306 = Array Size(array=w433) -> (size(s)=w435:i32[])
        n307 = Index Array(array=w435, index=0) -> (element=w432:i32)
        n308 = Greater?(x=w408, y=0) -> (0:w404:bool)
        n309 = for {
          N: w432 -> [_]
          tunnel: w433 -> [w476] mode=indexing
          shift-right: [w471] -> w429
          shift-left: 0 -> [w472]
          # "Caso numero 4"
          n310 = local read "Usuario nuevo 2"() -> (w474:string)
          n311 = Index Array(array=w476, index=0) -> (element=w475:string)
          n312 = Equal?(x=w475, y=w474) -> (x = y?=w473:bool)
          n313 = case shown="True" w473 {
            tunnel: w472 -> [w478 w480]
            tunnel: [w478 w479] -> w471
            frame False {
            }
            frame True {
              n314 = local read "Usuario nuevo 2"() -> (w481:string)
              n315 = Concatenate Strings("Usuario \"", w481, "\" existe en la base de datos.\nNo se puede agregar nuevamente." ("message")) -> (w483:string)
              n316 = Increment(x=w480) -> (x+1=w479:i32)
              n317 = One Button Dialog(message=w483) -> ()  [unwired: 1 in, 1 out]
            }
          }
        }
        n318 = local read "Contraseña nueva 2"() -> (w431:string)
        n319 = local read "Usuario nuevo 2"() -> (w430:string)
        n320 = Equal?(x=w430, y=w431) -> (x = y?=w398:bool)
        n321 = case shown="True" w398 {
          tunnel: w429 -> [w467 w468]
          tunnel: [w467 w469] -> w424
          frame False {
          }
          frame True {
            # "Caso numero 2"
            n322 = Increment(x=w468) -> (x+1=w469:i32)
            n323 = One Button Dialog(message="La contraseña debe ser diferente al usuario!") -> ()  [unwired: 1 in, 1 out]
          }
        }
        n324 = local read "Contraseña nueva 2"() -> (w422:string)
        n325 = String Length(string=w422) -> (length=w423:i32)
        n326 = Greater Or Equal?(x=w423, y=8) -> (x >= y?=w426:bool)
        n327 = Less Or Equal?(x=w423, y=16) -> (x <= y?=w425:bool)
        n328 = And(x=w426, y=w425) -> (x .and. y?=w421:bool)
        n329 = case shown="False" w421 {
          tunnel: w424 -> [w463 w466]
          tunnel: [w465 w466] -> w418
          frame False {
            n330 = Increment(x=w463) -> (x+1=w465:i32)
            n331 = One Button Dialog(message="La contraseña debe de tener\nentre 8 y 16 caracteres.") -> ()  [unwired: 1 in, 1 out]
          }
          frame True {
          }
        }
        n332 = local read "Usuario nuevo 2"() -> (w417:string)
        n333 = String Length(string=w417) -> (length=w420:i32)
        n334 = Greater?(x=w420, y=0) -> (0:w416:bool)
        n335 = case shown="False" w416 {
          tunnel: w418 -> [w461 w462]
          tunnel: [w460 w462] -> w412
          frame False {
            n336 = Increment(x=w461) -> (x+1=w460:i32)
            n337 = One Button Dialog(message="Favor ingresar el \nusuario en el campo\n\"Usuario nuevo\"") -> ()  [unwired: 1 in, 1 out]
          }
          frame True {
          }
        }
        n338 = local read "Contraseña nueva 2"() -> (w410:string)
        n339 = Match Pattern(string=w410, regular expression="[a-z]") -> (offset past match=w414:i32)  [unwired: 1 in, 3 out]
        n340 = Greater?(x=w414, y=0) -> (0:w411:bool)
        n341 = case shown="False" w411 {
          tunnel: w412 -> [w455 w458]
          tunnel: [w457 w458] -> w406
          frame False {
            n342 = Increment(x=w455) -> (x+1=w457:i32)
            n343 = One Button Dialog(message="La contraseña debe de tener\ncomo minimo una letra\nminuscula.") -> ()  [unwired: 1 in, 1 out]
          }
          frame True {
          }
        }
        n344 = case shown="False" w404 {
          tunnel: w406 -> [w451 w454]
          tunnel: [w453 w454] -> w402
          frame False {
            n345 = Increment(x=w451) -> (x+1=w453:i32)
            n346 = One Button Dialog(message="La contraseña debe de tener\ncomo minimo una letra\nMayuscula.") -> ()  [unwired: 1 in, 1 out]
          }
          frame True {
          }
        }
        n347 = Equal?(x=w402, y=0) -> (x = y?=w401:bool)
        n348 = case shown="True" w401 {
          tunnel: ["" ""] -> w400
          tunnel: ["" ""] -> w399
          frame False {
            n349 = One Button Dialog(message="No se pudo ingresar el\nusuario a la base de \ndatos") -> ()  [unwired: 1 in, 1 out]
          }
          frame True {
            n350 = local read "Contraseña nueva 2"() -> (w443:string)
            n351 = local read "Usuario nuevo 2"() -> (w444:string)
            n352 = local read "Base de datos"() -> (w445:string[][])
            n353 = Build Array(w444, w443) -> (w448:string[])
            n354 = Build Array (concatenate)(w445, w448) -> (w449:string[][])
            n355 = Concatenate Strings("Usuario \"", w444, "\" agregado a la base de datos" ("message")) -> (w450:string)
            n356 = local write "Base de datos"(w449) -> ()
            n357 = One Button Dialog(message=w450) -> ()  [unwired: 1 in, 1 out]
          }
        }
        n358 = local write "Contraseña nueva 2"(w400) -> ()
        n359 = local write "Usuario nuevo 2"(w399) -> ()
      }
      event "Eliminar usuario 2": Value Change {
        # "Resultado de la Bandera:\n0: Usuario no existe en la base de datos.\n1: Usuario eliminado de la base de datos.\n2: No se puede eliminar el perfil \"admin\"."
        # "Bandera"
        # "Resultado de la Bandera:\n0: Usuario no existe en la base de datos.\n1: Usuario eliminado de la base de datos.\n2: No se puede eliminar el perfil \"admin\"."
        n360 = event-data() -> ("OldVal"=w494:bool)  [unwired: 1 in, 5 out]
        n361 = local read "Base de datos"() -> (w490:string[][])
        n362 = Array Size(array=w490) -> (size(s)=w493:i32[])
        n363 = local write "Eliminar usuario 2"(w494) -> ()
        n364 = Index Array(array=w493, index=0) -> (element=w491:i32)
        n365 = for {
          N: w491 -> [w521]
          tunnel: w490 -> [w524] mode=indexing
          shift-right: [w519] -> w486
          shift-left: 0 -> [w520]
          i -> [w522]
          n366 = local read "Usuario a eliminar 2"() -> (w517:string)
          n367 = Index Array(array=w524, index=0) -> (element=w518:string)
          n368 = Equal?(x=w518, y=w517) -> (x = y?=w523:bool)
          n369 = case shown="False" w523 {
            tunnel: w522 -> [_ w531]
            tunnel: w521 -> [_ w532]
            tunnel: w520 -> [w526 w529]
            tunnel: [w526 w527] -> w519
            tunnel: w518 -> [_ w530]
            frame False {
            }
            frame True {
              n370 = Equal?(x=w531, y=0) -> (x = y?=w533:bool)
              n371 = Increment(x=w529) -> (x+1=w528:i32)
              n372 = case shown="False" w533 {
                tunnel: w532 -> [w541 w554]
                tunnel: w531 -> [w540 _]
                tunnel: w530 -> [_ w556]
                tunnel: w528 -> [w535 w553]
                tunnel: [w535 w552] -> w527
                frame False {
                  n373 = local read "Base de datos"() -> (w542:string[][])
                  n374 = Delete From Array(array=w542, length=w541, index (row)=w540) -> (deleted portion=w537:string[][], array with subset deleted=w538:string[][])  [unwired: 1 in]
                  n375 = Array Size(array=w537) -> (size(s)=w544:i32[])
                  n376 = Index Array(array=w544, index=0) -> (element=w543:i32)
                  n377 = Decrement(x=w543) -> (x-1=w539:i32)
                  n378 = for {
                    N: w539 -> [_]
                    shift-right: [w546] -> w536
                    shift-left: w538 -> [w550]
                    tunnel: w537 -> [w549]
                    i -> [w551]
                    n379 = Increment(x=w551) -> (x+1=w548:i32)
                    n380 = Index Array(array=w549, index (row)=w548) -> (element=w547:string[])  [unwired: 1 in]
                    n381 = Build Array (concatenate)(w550, w547) -> (w546:string[][])
                  }
                  n382 = local write "Base de datos"(w536) -> ()
                }
                frame True {
                  n383 = local read "Usuario a eliminar 2"() -> (w557:string)
                  n384 = Equal?(x=w556, y=w557) -> (x = y?=w555:bool)
                  n385 = case shown="False" w555 {
                    tunnel: w554 -> [w559 _]
                    tunnel: w553 -> [w558 w564]
                    tunnel: [w558 w563] -> w552
                    frame False {
                      n386 = local read "Base de datos"() -> (w562:string[][])
                      n387 = Delete From Array(array=w562, length=w559, index (row)=1) -> (deleted portion=w561:string[][])  [unwired: 1 in, 1 out]
                      n388 = local write "Base de datos"(w561) -> ()
                    }
                    frame True {
                      n389 = Increment(x=w564) -> (x+1=w563:i32)
                      n390 = One Button Dialog(message="No se puede eliminar el perfir de \"admin\".") -> ()  [unwired: 1 in, 1 out]
                    }
                  }
                }
              }
            }
          }
        }
        n391 = Equal?(x=w486, y=0) -> (x = y?=w487:bool)
        n392 = case shown="False" w487 {
          tunnel: w486 -> [w497 _]
          tunnel: [w495 ""] -> w485
          frame False {
            n393 = Equal?(x=w497, y=1) -> (x = y?=w498:bool)
            n394 = case shown="True" w498 {
              tunnel: ["" ""] -> w495
              frame False {
                n395 = One Button Dialog(message="El perfil \"admin\" es el encargado\nde gestionar la base de datos, por\ntanto no se puede eliminar dicho\nperfil.") -> ()  [unwired: 1 in, 1 out]
              }
              frame True {
                n396 = local read "Usuario a eliminar 2"() -> (w502:string)
                n397 = local read "Usuario a eliminar 2"() -> (w507:string)
                n398 = local read "USUARIO"() -> (w503:string)
                n399 = Equal?(x=w502, y=w503) -> (x = y?=w501:bool)
                n400 = case shown="True" w501 {
                  frame False {
                  }
                  frame True {
                    n401 = local write "USUARIO"("") -> ()
                    n402 = local write "CONTRASEÑA"("") -> ()
                    n403 = local write "Tab control 1"(T1."Bienvenidos" ("Tab control")) -> ()
                  }
                }
                n404 = Concatenate Strings("Usuario \"", w507, "\" eliminado de la base de datos." ("message")) -> (w508:string)
                n405 = One Button Dialog(message=w508) -> ()  [unwired: 1 in, 1 out]
              }
            }
          }
          frame True {
            n406 = local read "Usuario a eliminar 2"() -> (w513:string)
            n407 = Concatenate Strings("Usuario \"", w513, "\" no existe en la base de datos." ("message")) -> (w516:string)
            n408 = One Button Dialog(message=w516) -> ()  [unwired: 1 in, 1 out]
          }
        }
        n409 = local write "Usuario a eliminar 2"(w485) -> ()
      }
      event "Terminar sesión admin 2": Value Change {
        n410 = event-data() -> ("OldVal"=w569:bool)  [unwired: 1 in, 5 out]
        n411 = local write "Terminar sesión admin 2"(w569) -> ()
        n412 = local write "USUARIO  2"("") -> ()
        n413 = local write "Tab control 2"(T1."Bienvenidos" ("Tab control")) -> ()
        n414 = local write "CONTRASEÑA 2"("") -> ()
      }
      event "Terminar sesión usuario 2": Value Change {
        # "Menú usuario 2"
        n415 = event-data() -> ("OldVal"=w571:bool)  [unwired: 1 in, 5 out]
        n416 = local write "Terminar sesión usuario 2"(w571) -> ()
        n417 = local write "Menu2"(enum32{"1", "2", "3", "4", "5", "6"}."1" ("Menu2")) -> ()
        n418 = local write "USUARIO  2"("") -> ()
        n419 = local write "Tab control 2"(T1."Bienvenidos" ("Tab control")) -> ()
        n420 = local write "CONTRASEÑA 2"("") -> ()
      }
      event "Secuencia de leds 2": Value Change {
        n421 = event-data() -> ("OldVal"=w576:bool)  [unwired: 1 in, 5 out]
        n422 = local write "Secuencia de leds 2"(w576) -> ()
        n423 = local write "Menu2"(enum32{"1", "2", "3", "4", "5", "6"}."2" ("Menu2")) -> ()
        n424 = flat-sequence {
          frame #0 {
            n425 = local read "Led1 2"() -> (w579:bool)
            n426 = Not(x=w579) -> (.not. x?=w578:bool)
            n427 = Wait (ms)(milliseconds to wait=u32 1000) -> ()  [unwired: 1 out]
            n428 = local write "Led1 2"(w578) -> ()
          }
          frame #1 {
            n429 = local read "Led2 2"() -> (w581:bool)
            n430 = Wait (ms)(milliseconds to wait=u32 1000) -> ()  [unwired: 1 out]
            n431 = Not(x=w581) -> (.not. x?=w582:bool)
            n432 = local write "Led2 2"(w582) -> ()
            n433 = local write "Led1 2"(FALSE ("Led1")) -> ()
          }
          frame #2 {
            n434 = local read "Led3 2"() -> (w586:bool)
            n435 = Wait (ms)(milliseconds to wait=u32 1000) -> ()  [unwired: 1 out]
            n436 = Not(x=w586) -> (.not. x?=w585:bool)
            n437 = local write "Led3 2"(w585) -> ()
            n438 = local write "Led2 2"(FALSE ("Led1")) -> ()
          }
          frame #3 {
            n439 = local read "Led4 2"() -> (w590:bool)
            n440 = Wait (ms)(milliseconds to wait=u32 1000) -> ()  [unwired: 1 out]
            n441 = Not(x=w590) -> (.not. x?=w591:bool)
            n442 = local write "Led4 2"(w591) -> ()
            n443 = local write "Led3 2"(FALSE ("Led1")) -> ()
          }
          frame #4 {
            n444 = local read "Led5 2"() -> (w593:bool)
            n445 = Wait (ms)(milliseconds to wait=u32 1000) -> ()  [unwired: 1 out]
            n446 = Not(x=w593) -> (.not. x?=w592:bool)
            n447 = local write "Led5 2"(w592) -> ()
            n448 = local write "Led4 2"(FALSE ("Led1")) -> ()
          }
          frame #5 {
            n449 = local read "Led6 2"() -> (w598:bool)
            n450 = Wait (ms)(milliseconds to wait=u32 1000) -> ()  [unwired: 1 out]
            n451 = Not(x=w598) -> (.not. x?=w599:bool)
            n452 = local write "Led6 2"(w599) -> ()
            n453 = local write "Led5 2"(FALSE ("Led1")) -> ()
          }
          frame #6 {
            n454 = local read "Led7 2"() -> (w602:bool)
            n455 = Wait (ms)(milliseconds to wait=u32 1000) -> ()  [unwired: 1 out]
            n456 = Not(x=w602) -> (.not. x?=w601:bool)
            n457 = local write "Led7 2"(w601) -> ()
            n458 = local write "Led6 2"(FALSE ("Led1")) -> ()
          }
          frame #7 {
            n459 = local read "Led8 2"() -> (w605:bool)
            n460 = Wait (ms)(milliseconds to wait=u32 1000) -> ()  [unwired: 1 out]
            n461 = Not(x=w605) -> (.not. x?=w606:bool)
            n462 = local write "Led8 2"(w606) -> ()
            n463 = local write "Led7 2"(FALSE ("Led1")) -> ()
          }
          frame #8 {
            n464 = Wait (ms)(milliseconds to wait=u32 1000) -> ()  [unwired: 1 out]
            n465 = local write "Led8 2"(FALSE ("Led1")) -> ()
          }
        }
      }
      event "Gráfica del seno 2": Value Change {
        # "Gráfica del seno"
        # "Este bloque\nrecibe un cluster"
        # "Para mostrar la gráfoca en x,  y"
        n466 = event-data() -> ("OldVal"=w611:bool)  [unwired: 1 in, 5 out]
        n467 = local write "Gráfica del seno 2"(w611) -> ()
        n468 = local write "Menu2"(enum32{"1", "2", "3", "4", "5", "6"}."3" ("Menu2")) -> ()
        n469 = Multiply(x=200.0, y=3.141592653589793) -> (x*y=w617:dbl)
        n470 = for {
          N: w617 -> [_]
          tunnel: [w619] -> w613 mode=indexing
          tunnel: [w618] -> w614 mode=indexing
          i -> [w622]
          # "x"
          # "y"
          n471 = Wait (ms)(milliseconds to wait=u32 1) -> ()  [unwired: 1 out]
          n472 = Divide(x=w622, y=100) -> (x/y=w618:dbl)
          n473 = Sine(x=w618) -> (sin(x)=w619:dbl)
        }
        n474 = Bundle(w614, w613) -> (→"Gráfica del seno 2":cluster{dbl[], dbl[]})  [unwired: 1 in]
      }
      event "Circulo de la muerte 2": Value Change {
        n475 = event-data() -> ("OldVal"=w624:bool)  [unwired: 1 in, 5 out]
        n476 = local write "Circulo de la muerte 2"(w624) -> ()
        n477 = local write "Menu2"(enum32{"1", "2", "3", "4", "5", "6"}."4" ("MenuU")) -> ()
        n478 = for {
          N: 100 -> [_]
          tunnel: [w631] -> w627 mode=indexing
          tunnel: [w629] -> w626 mode=indexing
          i -> [w630]
          n479 = Multiply(x=0.3183098861837907, y=w630) -> (x*y=w633:dbl)
          n480 = Sine & Cosine(0:w633) -> (1:w632:dbl, 2:w629:dbl)
          n481 = Multiply(x=w632, y=w630) -> (x*y=w631:dbl)
        }
        n482 = Bundle(w627, w626) -> (→"Circulo de muerte 2":cluster{dbl[], dbl[]})  [unwired: 1 in]
      }
      event "Llenado de un tanque 2": Value Change {
        n483 = event-data() -> ("OldVal"=w637:bool)  [unwired: 1 in, 5 out]
        n484 = local write "Circulo de la muerte 2"(w637) -> ()
        n485 = local write "Menu2"(enum32{"1", "2", "3", "4", "5", "6"}."5" ("MenuU")) -> ()
        n486 = for {
          N: 100 -> [_]
          i -> [w639]
          n487 = Wait (ms)(milliseconds to wait=u32 100) -> ()  [unwired: 1 out]
          "tanque de chamber" <- w639
        }
      }
      event "Hora y fecha actual 2": Value Change {
        # "Hora"
        # "Fecha"
        n488 = event-data() -> ("OldVal"=w652:bool)  [unwired: 1 in, 5 out]
        n489 = local write "Hora y fecha actual 2"(w652) -> ()
        n490 = local write "Menu2"(enum32{"1", "2", "3", "4", "5", "6"}."6" ("MenuU")) -> ()
        n491 = Get Date/Time In Seconds() -> (seconds since 1Jan1904=w651:timestamp)
        n492 = Get Date/Time In Seconds() -> (seconds since 1Jan1904=w641:timestamp)
        n493 = Get Date/Time String(seconds (now)=w651) -> (date string=w650:string)  [unwired: 2 in, 1 out]
        n494 = Get Date/Time String(seconds (now)=w641) -> (time string=w640:string)  [unwired: 2 in, 1 out]
        n495 = Concatenate Strings("Fecha:" ("date string"), "\n", "\n", w650) -> (→"Fecha 2":string)
        n496 = Concatenate Strings("Hora:" ("date string"), "\n", "\n", w640) -> (→"Hora 2":string)
      }
    }
  }
  "Led1" <- FALSE ("Led1")
  "Led2" <- FALSE ("Led2")
  "Led3" <- FALSE ("Led3")
  "Led4" <- FALSE ("Led4")
  "Led5" <- FALSE ("Led5")
  "Led6" <- FALSE ("Led6")
  "Led7" <- FALSE ("Led7")
  "Led8" <- FALSE ("Led8")
  "Led1 2" <- FALSE ("Led1 2")
  "Led2 2" <- FALSE ("Led2 2")
  "Led3 2" <- FALSE ("Led3 2")
  "Led4 2" <- FALSE ("Led4 2")
  "Led5 2" <- FALSE ("Led5 2")
  "Led6 2" <- FALSE ("Led6 2")
  "Led7 2" <- FALSE ("Led7 2")
  "Led8 2" <- FALSE ("Led8 2")
